vi "Get TCP Connection ref.vi"(11 "TCP Process in":refnum<class "TCP Process.lvclass">) -> (2 "TCP Connection ref":refnum<k5>, 3 "TCP Process out":refnum<class "TCP Process.lvclass">)   [LabVIEW 2019, in "TimingDRV Engine.lvlib" / "TCP Process.lvclass"]
uses:
  TCP Process.lvclass
  TCP Process.lvclass/TCP Process.ctl
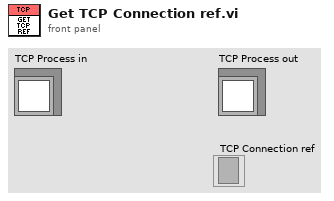
[diagram p1: front panel]
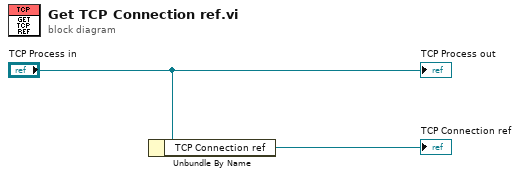
[diagram p0: block diagram]
diagram:
  n1 = Unbundle By Name("TCP Process in") -> ("TCP Connection ref"=→"TCP Connection ref":refnum<k5>)
  "TCP Process out" <- "TCP Process in"
